vi "MenuBar.vi"(8 "ErrI":errorcluster) -> (0 "ErrO":errorcluster)   [LabVIEW 2020]
doc: "Use this template to create a dialog box with event handling."
uses:
  <vilib>/Utility/cursorutil.llb/Set Cursor (Cursor ID).vi
panel:
  in  "User":bool
  in  "StopTest":bool
  in  "StartTest":bool
  in  "Exit":bool
  in  "OK":bool
  out "Slide":dbl(slide) scale=0.0..10.0
  out "Status":string
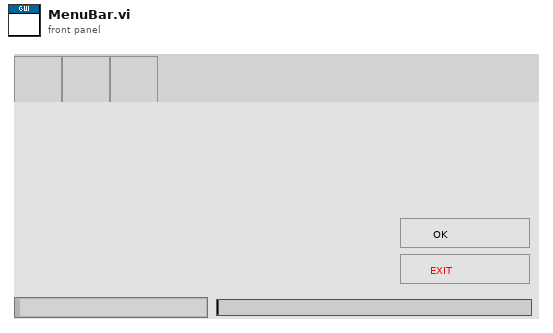
[diagram p1: front panel]
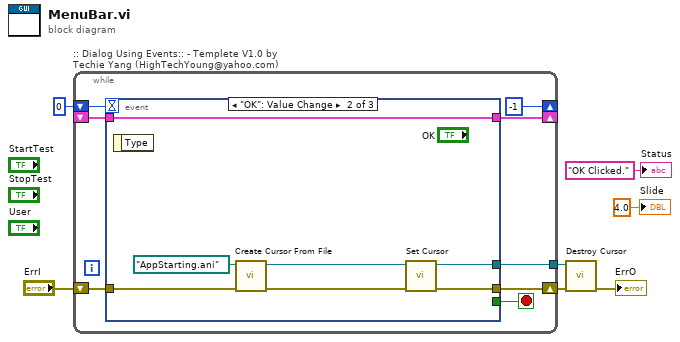
[diagram p0: block diagram]
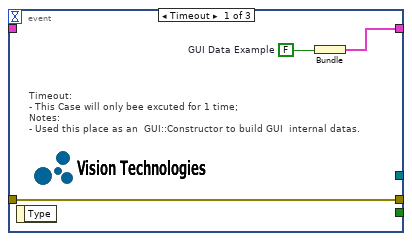
[diagram p2: hidden frame]
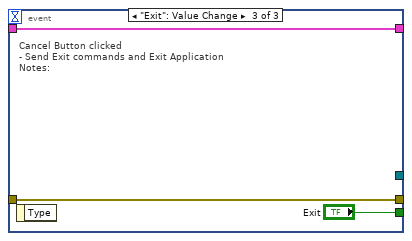
[diagram p3: hidden frame]
diagram:
  n1 = while ":: Dialog Using Events:: - Templete V1.0 by Techie Yang (HighTechYoung@yahoo.com)" {
    shift-right: [w12] -> w3
    shift-left: "ErrI" -> [w11]
    shift-right: [w14] -> _
    shift-left: _ -> [w13]
    shift-right: [-1] -> _
    shift-left: 0 -> [w9]
    tunnel: [w8] -> w1
    stop <- w15 stop-if-true
    n2 = event shown="[1] \"OK\": Value Change" {
      selector: _ -> [_ _ _]
      dyn-events: _ -> [_ _ _]
      timeout: w9 -> [_ _ _]
      tunnel: [_ _ "Exit"] -> w15
      tunnel: w11 -> [w18 w21 w27]
      tunnel: [w18 w20 w27] -> w12
      tunnel: [w16 w25 w28] -> w14
      tunnel: w13 -> [_ w25 w28]
      tunnel: [_ w19 _] -> w8
      event Timeout {
        w17 = FALSE  # GUI Data Example
        # "Timeout:\n- This Case will only bee excuted for 1 time;\nNotes:\n- Used this place as an  GUI::Constructor to build GUI  internal datas."
        n3 = event-data() -> ()  [unwired: 2 out]
        n4 = Bundle("GUI Data Example"=w17) -> (w16:cluster{"GUI Data Example":bool})  [unwired: 1 in]
      }
      event "OK": Value Change {
        n5 = event-data() -> ()  [unwired: 2 out]
        n6 = call <vilib>:"Create Cursor From File.vi"("error in (no error)"=w21, "cursor file"=path "AppStarting.ani") -> ("error out"=w23:errorcluster, "cursor ID"=w22:refnum<k1>)  [unwired: 8 in]
        n7 = call-poly <vilib>:"Set Cursor.vi"("error in (no error)"=w23, "cursor ID"=w22) -> ("error out"=w20:errorcluster, "previous cursor ID"=w19:refnum<k1>)  [unwired: 8 in]
      }
      event "Exit": Value Change {
        # "Cancel Button clicked\n- Send Exit commands and Exit Application\nNotes:"
        n8 = event-data() -> ()  [unwired: 2 out]
      }
    }
  }
  n9 = call <vilib>:"Destroy Cursor.vi"("cursor ID"=w1, "error in (no error)"=w3) -> ("error out"=→"ErrO":errorcluster)  [unwired: 8 in]
  "Status" <- "OK Clicked." ("Status")
  "Slide" <- 4.0 ("Slide")
